vi "GenNodes.vi"() -> (3 "Array":i32[][](array[numeric]))   [LabVIEW 2020]
panel:
  out "element":i32
  in  "index (row)":i32
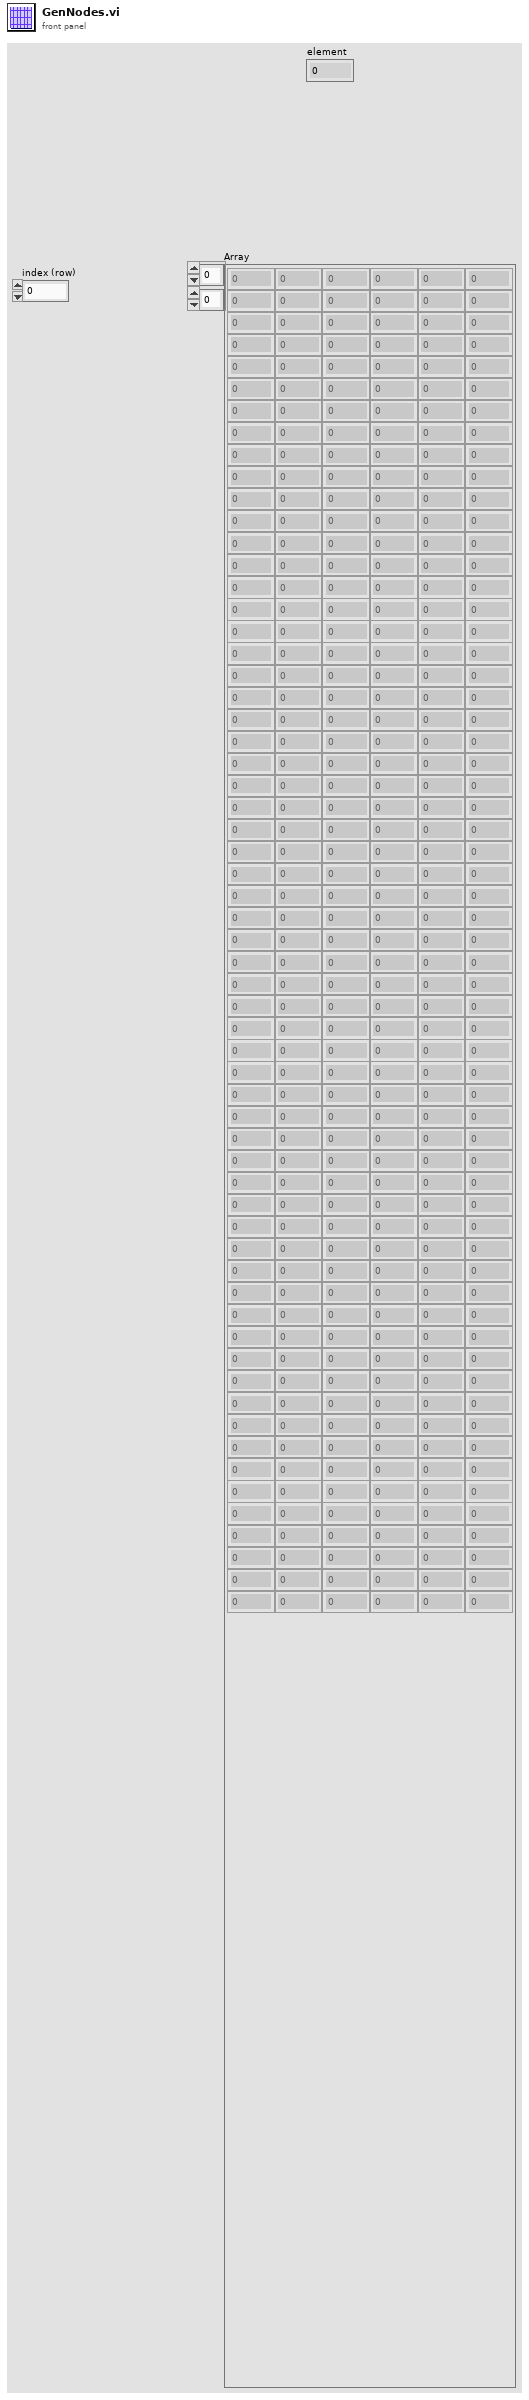
[diagram p1: front panel]
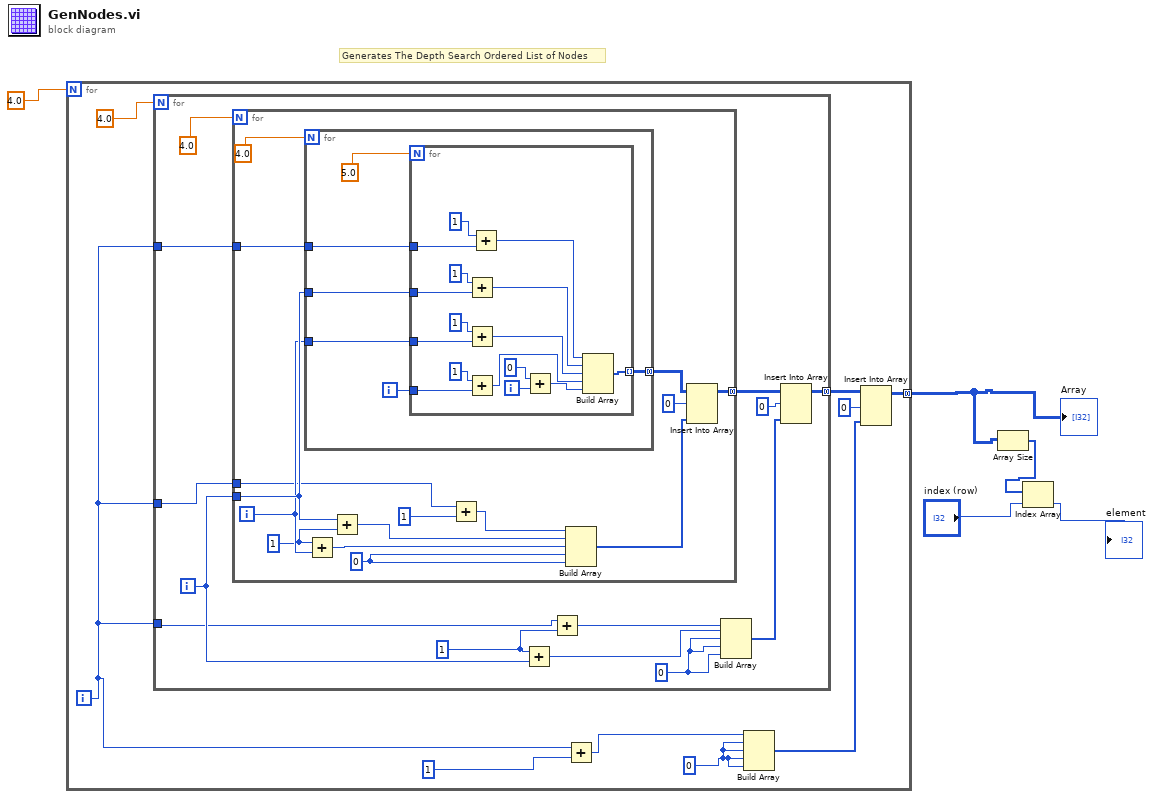
[diagram p0: block diagram]
diagram:
  # "Generates The Depth Search Ordered List of Nodes"
  n1 = for {
    N: 4.0 -> [_]
    tunnel: [w7] -> w3 mode=concatenating
    i -> [w12]
    w13 = 0
    n2 = for {
      N: 4.0 -> [_]
      tunnel: [w27] -> w10 mode=concatenating
      tunnel: w12 -> [w19]
      tunnel: w12 -> [w18]
      tunnel: w12 -> [w17]
      i -> [w23]
      w15 = 1
      w20 = 0
      n3 = for {
        N: 4.0 -> [_]
        tunnel: w23 -> [w38]
        tunnel: [w40] -> w21 mode=concatenating
        tunnel: w19 -> [w31]
        tunnel: w18 -> [w30]
        i -> [w36]
        w33 = 0
        w35 = 1
        n4 = for {
          N: 4.0 -> [_]
          tunnel: w38 -> [w48]
          tunnel: w36 -> [w47]
          tunnel: [w46] -> w41 mode=concatenating
          tunnel: w31 -> [w43]
          i -> [w45]
          n5 = for {
            N: 5.0 -> [_]
            tunnel: w48 -> [w63]
            tunnel: w47 -> [w60]
            tunnel: [w64] -> w46 mode=indexing
            tunnel: w45 -> [w54]
            tunnel: w43 -> [w51]
            i -> [w56]
            n6 = Add(x=1, y=w63) -> (x+y=w61:i32)
            n7 = Add(x=1, y=w60) -> (x+y=w58:i32)
            n8 = Add(x=1, y=w54) -> (x+y=w53:i32)
            n9 = Add(x=1, y=w51) -> (x+y=w49:i32)
            n10 = Add(x=0, y=w56) -> (x+y=w55:i32)
            n11 = Build Array(w49, w61, w58, w53, w55) -> (w64:i32[])
          }
        }
        n12 = Add(x=w35, y=w36) -> (x+y=w34:i32)
        n13 = Add(x=w38, y=w35) -> (x+y=w37:i32)
        n14 = Add(x=w30, y=1) -> (x+y=w29:i32)
        n15 = Build Array(w29, w37, w34, w33, w33) -> (w39:i32[])
        n16 = Insert Into Array(array=w41, index (row)=0, new element=w39) -> (w40:i32[][])  [unwired: 1 in]
      }
      n17 = Add(x=w15, y=w23) -> (x+y=w22:i32)
      n18 = Add(x=w17, y=w15) -> (x+y=w16:i32)
      n19 = Build Array(w16, w22, w20, w20, w20) -> (w26:i32[])
      n20 = Insert Into Array(array=w21, index (row)=0, new element=w26) -> (w27:i32[][])  [unwired: 1 in]
    }
    n21 = Add(x=w12, y=1) -> (x+y=w11:i32)
    n22 = Build Array(w11, w13, w13, w13, w13) -> (w9:i32[])
    n23 = Insert Into Array(array=w10, index (row)=0, new element=w9) -> (w7:i32[][])  [unwired: 1 in]
  }
  "Array" <- w3
  n24 = Array Size(array=w3) -> (size(s)=w2:i32[])
  n25 = Index Array(array=w2, index="index (row)") -> (element=→"element":i32)
